vi "testOpen.vi"() -> ()   [LabVIEW 2010]
uses:
  GlobalSpectHdl.vi
  GlobalCamOpen.vi
panel:
  out "camera opened":bool
  out "spectrometer opened":bool
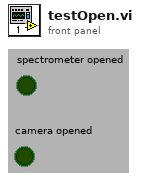
[diagram p1: front panel]
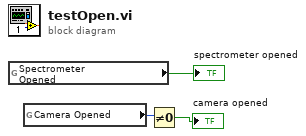
[diagram p0: block diagram]
diagram:
  n1 = global read "GlobalSpectHdl.vi" "Spectrometer \nOpened"() -> (→"spectrometer opened":bool)
  n2 = global read "GlobalCamOpen.vi" "Camera Opened"() -> (w1:u32)
  n3 = Not Equal To 0?(x=w1) -> (x != 0?=→"camera opened":bool)
